vi "Valve_Sim_Init.vi"(0 "object in":refnum<class "Valve_Sim.lvclass">, 5 "error in (no error)":errorcluster) -> (14 "object out":refnum<class "Valve_Sim.lvclass">, 19 "error out":errorcluster)   [LabVIEW 2024, in "Valve_Sim.lvclass"]
uses:
  Valve_Sim.lvclass
  Valve_Sim.lvclass/Valve_Sim.ctl
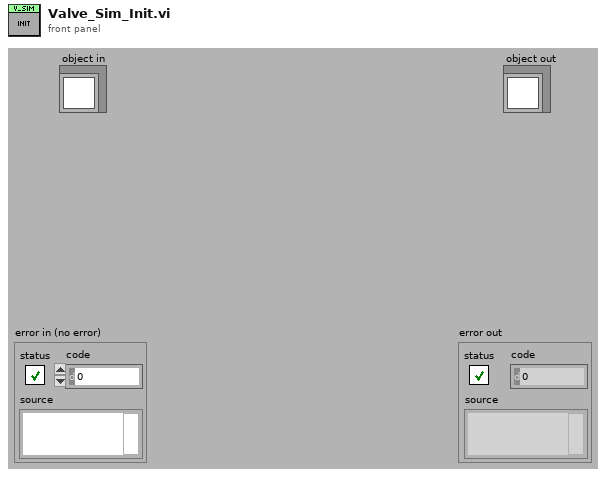
[diagram p1: front panel]
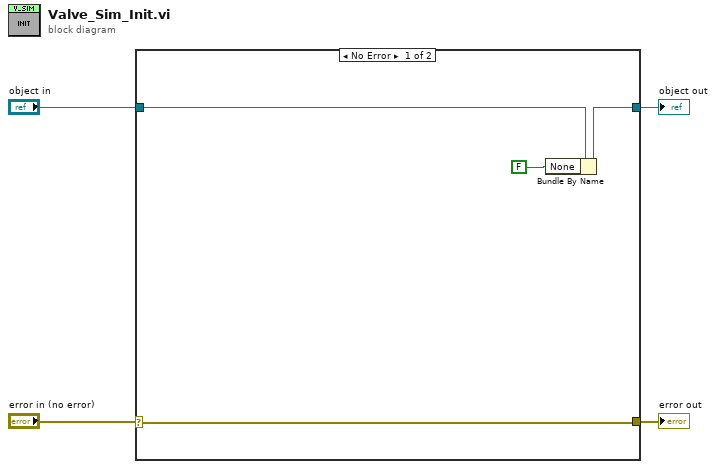
[diagram p0: block diagram]
diagram:
  n1 = case shown="No Error" "error in (no error)" {
    selector: "error in (no error)" -> [w6 w9]
    tunnel: [w8 w10] -> w4
    tunnel: "object in" -> [w5 w10]
    tunnel: [w6 w9] -> w1
    frame No Error {
      n2 = Bundle By Name(cluster=w5, "None"=FALSE) -> (w8:refnum<class "Valve_Sim.lvclass">)
    }
    frame Error {
    }
  }
  "object out" <- w4
  "error out" <- w1
